vi "Measure.vi"(8 "error in":errorcluster, 11 "PRM in":refnum<class "PRM.lvclass">) -> (0 "error out":errorcluster, 3 "PRM out":refnum<class "PRM.lvclass">)   [LabVIEW 2019, in "PRM.lvlib" / "PRM.lvclass"]
uses:
  Library/PRM.lvclass
  C:/Users/Public/Documents/Development/builds/Instruments/Instruments.lvlibp/Library/Instruments.lvclass
  builds/Instruments/Instruments.lvlibp/Accessors/Read dt.vi
  builds/Instruments/Instruments.lvlibp/Accessors/Write Measured.vi
  builds/Instruments/Instruments.lvlibp/Library/Instruments.lvclass
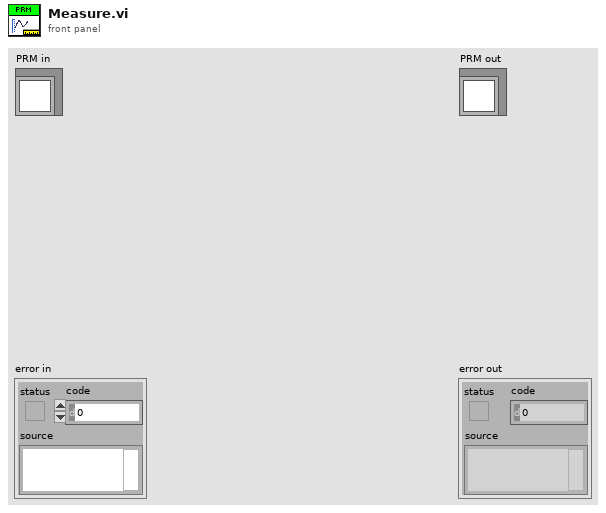
[diagram p1: front panel]
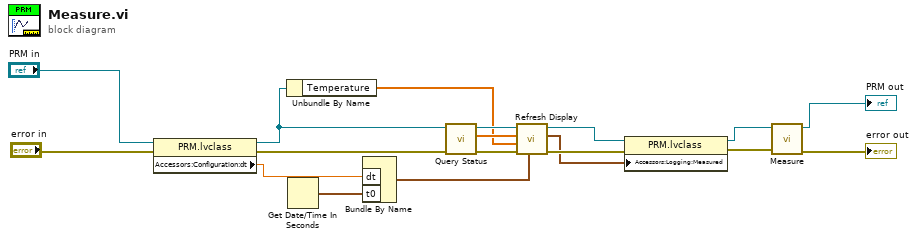
[diagram p0: block diagram]
diagram:
  n1 = property class="PRM.lvclass"(reference="PRM in", error in="error in") -> (reference out=w2:refnum<class "PRM.lvclass">, error out=w12:errorcluster, "Accessors:Configuration:dt"=w15:dbl)
  n2 = Unbundle By Name(w2) -> ("Temperature"=w1:dbl[])
  n3 = Get Date/Time In Seconds() -> (seconds since 1Jan1904=w13:timestamp)
  n4 = Bundle By Name("dt"=w15, "t0"=w13) -> (w4:waveform(dbl))  [unwired: 1 in]
  n5 = call-dynamic "Query Status.vi"("error in (no error)"=w12, "PRM in"=w2) -> ("error out"=w8:errorcluster, "Resistance"=w3:dbl[], "PRM out"=w9:refnum<class "PRM.lvclass">)  [unwired: 7 in]
  n6 = call "Refresh Display.vi"("WaveformTemplate"=w4, "error in"=w8, "Temperature"=w1, "Resistance"=w3, "PRM in"=w9) -> ("error out"=w6:errorcluster, "Measured"=w5:waveform(dbl)[], "PRM out"=w7:refnum<class "PRM.lvclass">)  [unwired: 4 in]
  n7 = property class="PRM.lvclass"(reference=w7, error in=w6, "Accessors:Logging:Measured"=w5) -> (reference out=w10:refnum<class "PRM.lvclass">, error out=w11:errorcluster)
  n8 = call-parent "Measure.vi"("error in"=w11, "Instruments in"=w10) -> ("error out"=→"error out":errorcluster, "Instruments out"=→"PRM out":refnum<class "PRM.lvclass">)  [unwired: 8 in]
